vi "Main.vi"() -> ()   [LabVIEW 2013]
uses:
  <vilib>/myRIO/Instrument Drivers/Onboard IO/I2C/vis/Smart Open.vi
  <vilib>/myRIO/Instrument Drivers/Onboard IO/I2C/vis/Configure.vi
  <vilib>/myRIO/Instrument Drivers/Onboard IO/I2C/vis/Write Read.vi
  <vilib>/myRIO/Instrument Drivers/Onboard IO/I2C/vis/Write.vi
  <vilib>/myRIO/Instrument Drivers/Onboard IO/DIO/vis/Smart Open.vi
  <vilib>/myRIO/Instrument Drivers/Onboard IO/DIO/vis/Read.vi
  <vilib>/myRIO/Instrument Drivers/Onboard IO/I2C/vis/Read.vi
  <vilib>/myRIO/Common/Instrument Driver Framework/myRIO v1.0/UART/vis/myRIO v1.0 Close UART.vi
  <vilib>/myRIO/Instrument Drivers/Onboard IO/I2C/vis/Open.vi
  <vilib>/myRIO/Instrument Drivers/Onboard IO/DIO/vis/Open.vi
  <vilib>/myRIO/Common/Instrument Driver Framework/myRIO v1.0/I2C/vis/myRIO v1.1 Open I2C.vi
  <vilib>/myRIO/Common/Instrument Driver Framework/myRIO v1.0/DIO/vis/myRIO v1.1 Open DIO.vi
  <vilib>/myRIO/Common/Instrument Driver Framework/Utilities/vis/Validate Channels.vi
  <vilib>/myRIO/Common/Instrument Driver Framework/myRIO v1.0/I2C/vis/myRIO v1.0 Reserve I2C.vi
  <vilib>/myRIO/Common/Instrument Driver Framework/myRIO v1.0/DIO/vis/myRIO v1.0 Reserve DIO.vi
  <vilib>/myRIO/Common/Instrument Driver Framework/myRIO v1.0/I2C/vis/myRIO v1.0 Build MUX Configuration I2C.vi
  <vilib>/myRIO/Common/Instrument Driver Framework/myRIO v1.0/Resource Manager/vis/myRIO v1.0 Reserve Channel List.vi
  <vilib>/myRIO/Common/Instrument Driver Framework/myRIO v1.0/DIO/vis/myRIO v1.0 Build MUX Configuration DIO.vi
  <vilib>/myRIO/Common/Instrument Driver Framework/myRIO v1.0/Resource Manager/vis/myRIO v1.0 Create Configuration List.vi
  <vilib>/myRIO/Common/Instrument Driver Framework/myRIO v1.0/Resource Manager/vis/myRIO v1.0 Reserve Channel.vi
  <vilib>/myRIO/Common/Instrument Driver Framework/myRIO v1.0/Resource Manager/vis/myRIO v1.0 Unreserve Channel.vi
  <vilib>/myRIO/Common/Instrument Driver Framework/myRIO v1.0/Resource Manager/vis/myRIO v1.0 Build Mutex Name.vi
  <vilib>/myRIO/Common/Instrument Driver Framework/myRIO v1.0/myRIO v1.1 Open.vi
  <vilib>/Utility/VariantDataType/GetNumericInfo.vi
  <vilib>/Utility/error.llb/Error Cluster From Error Code.vi
  <vilib>/myRIO/Common/Instrument Driver Framework/Utilities/vis/IO Manager.vi
  <vilib>/myRIO/Common/Instrument Driver Framework/Utilities/vis/Configuration Manager.vi
  <vilib>/myRIO/Common/Instrument Driver Framework/myRIO v1.0/Resource Manager/vis/myRIO v1.0 Configure IO.vi
  <vilib>/myRIO/Common/Instrument Driver Framework/myRIO v1.0/myRIO v1.0 Close.vi
  <vilib>/myRIO/Common/Instrument Driver Framework/myRIO v1.0/I2C/vis/myRIO v1.0 Configure I2C.vi
  <vilib>/myRIO/Common/Instrument Driver Framework/myRIO v1.0/I2C/vis/myRIO v1.0 Write I2C.vi
  <vilib>/myRIO/Common/Instrument Driver Framework/myRIO v1.0/I2C/vis/myRIO v1.0 Read I2C.vi
  <vilib>/myRIO/Common/Instrument Driver Framework/myRIO v1.0/DIO/vis/myRIO v1.0 Read DIO.vi
  <vilib>/myRIO/Common/Instrument Driver Framework/Utilities/vis/FPGA Ref Manager.vi
  <vilib>/myRIO/Common/Instrument Driver Framework/myRIO v1.0/myRIO v1.0 Reset FPGA.vi
  <vilib>/myRIO/Instrument Drivers/Utilities/Utilities.lvlib
panel:
  out "Thyst (hysteresis)":u8[](array[numeric]) format="%02x"
  out "Tset (limit set)":u8[](array[numeric]) format="%02x"
  out "Config":u8[](array[numeric]) format="%08b"
  out "alert":bool
  out "temperature [ºC]":dbl(slide) scale=20.0..30.0
  out "Ta (ambient temp)":u8[](array[numeric]) format="%02x"
  in  "[ESC]":bool
  # "Temperature Sensor demo"
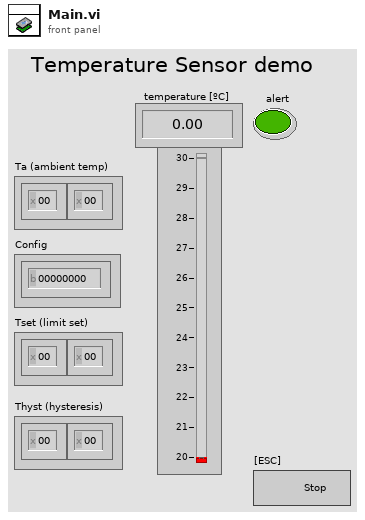
[diagram p1: front panel]
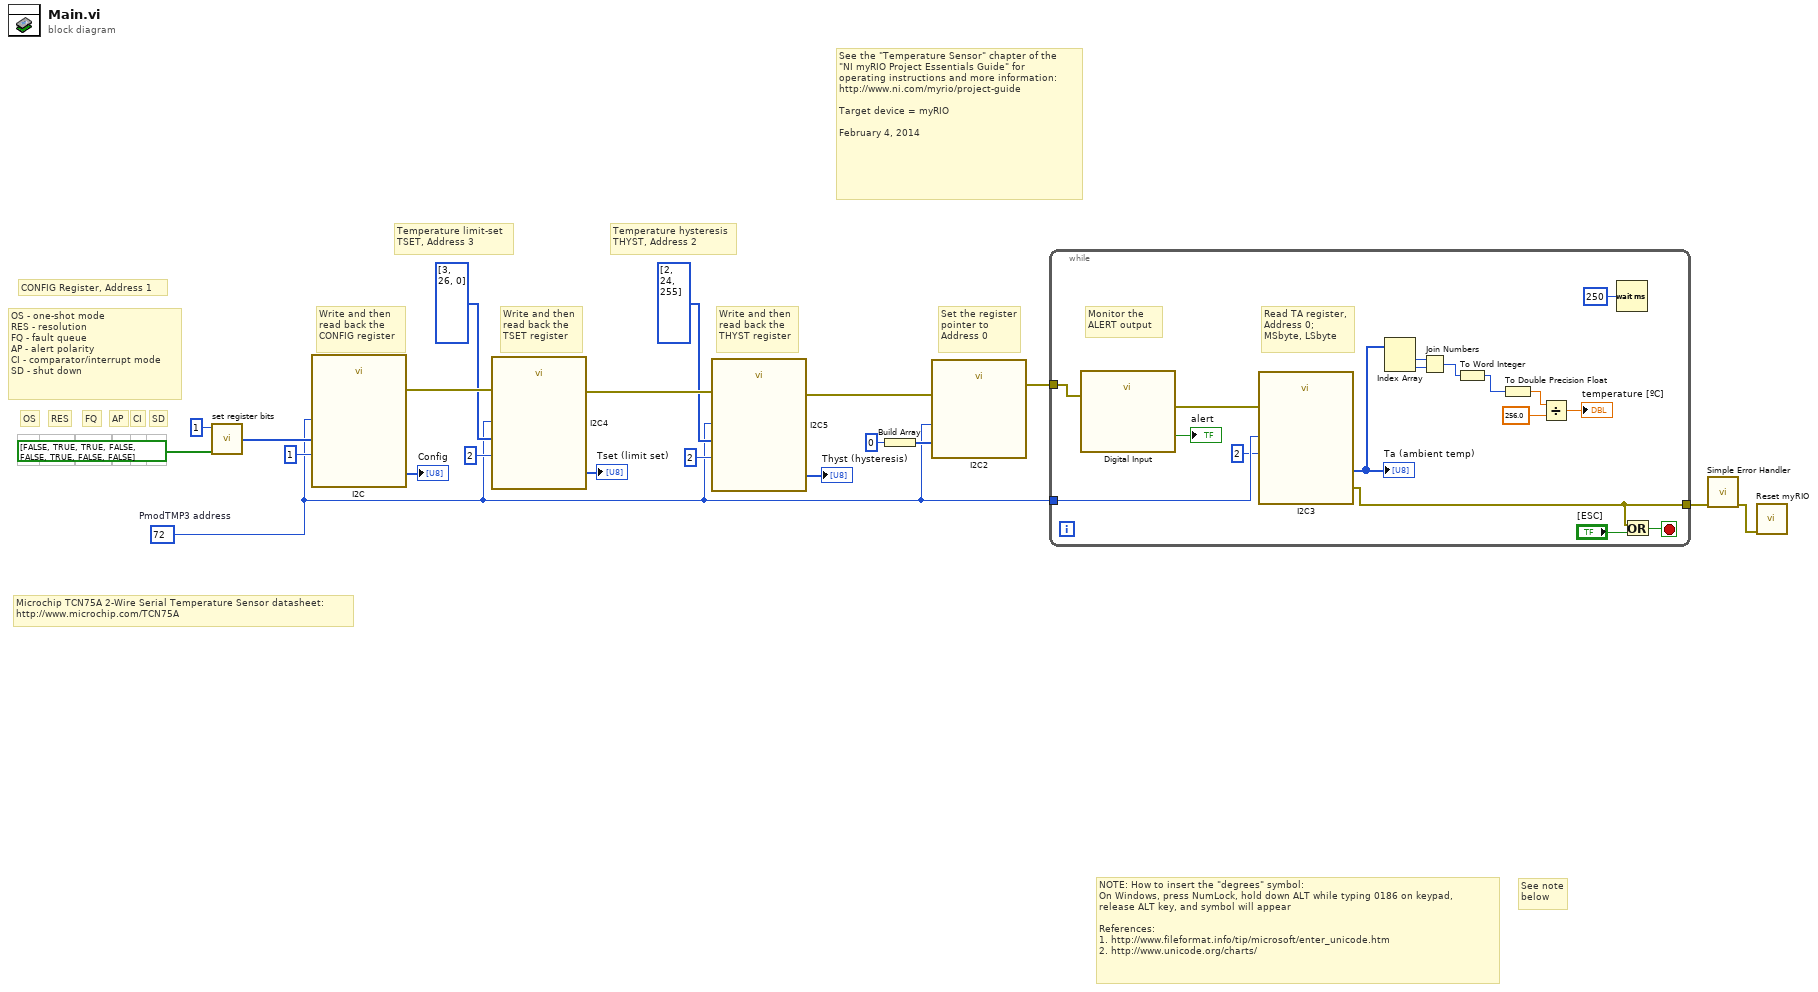
[diagram p0: block diagram]
diagram:
  w1 = u8 72  # PmodTMP3 address
  # "See the \"Temperature Sensor\" chapter of the\n\"NI myRIO Project Essentials Guide\" for\noperating instructions and more information: \nhttp://www.ni.com/myrio/project-guide\n\nTarget device = myRIO\n\nFebruary 4, 2014"
  # "Microchip TCN75A 2-Wire Serial Temperature Sensor datasheet:\nhttp://www.microchip.com/TCN75A"
  # "See note\nbelow"
  # "Write and then\nread back the\nCONFIG register"
  # "Write and then\nread back the\nTHYST register"
  # "Write and then\nread back the\nTSET register"
  # "Set the register\npointer to\nAddress 0"
  # "Temperature hysteresis\nTHYST, Address 2"
  # "Temperature limit-set\nTSET, Address 3"
  # "OS - one-shot mode\nRES - resolution\nFQ - fault queue\nAP - alert polarity\nCI - comparator/interrupt mode\nSD - shut down"
  # "SD"
  # "CI"
  # "AP"
  # "FQ"
  # "RES"
  # "OS"
  # "CONFIG Register, Address 1"
  # "NOTE: How to insert the \"degrees\" symbol:\nOn Windows, press NumLock, hold down ALT while typing 0186 on keypad,\nrelease ALT key, and symbol will appear\n\nReferences:\n1. http://www.fileformat.info/tip/microsoft/enter_unicode.htm\n2. http://www.unicode.org/charts/"
  n1 = call "set register bits.vi"("address"=u8 1, "register bits"=bool[] [FALSE, TRUE, TRUE, FALSE, FALSE, TRUE, FALSE, FALSE]) -> ("address / value"=w11:u8[])  [unwired: 5 in]
  n2 = call "I2C"("Slave Address (7-bit)"=w1, "Bytes to Write"=w11, "Byte Count"=u32 1) -> ("Bytes Read"=→"Config":u8[], "error out"=w15:errorcluster)  [unwired: 23 in]
  n3 = call "I2C4"("Slave Address (7-bit)"=w1, "Bytes to Write"=u8[] [3, 26, 0], "Byte Count"=u32 2, "error in (no error)"=w15) -> ("Bytes Read"=→"Tset (limit set)":u8[], "error out"=w14:errorcluster)  [unwired: 22 in]
  n4 = call "I2C5"("Slave Address (7-bit)"=w1, "Bytes to Write"=u8[] [2, 24, 255], "Byte Count"=u32 2, "error in (no error)"=w14) -> ("Bytes Read"=→"Thyst (hysteresis)":u8[], "error out"=w2:errorcluster)  [unwired: 22 in]
  n5 = Build Array(u8 0 ("address")) -> (w3:u8[])
  n6 = call "I2C2"("Slave Address (7-bit)"=w1, "Bytes to Write"=w3, "error in (no error)"=w2) -> ("error out"=w18:errorcluster)  [unwired: 24 in]
  n7 = while {
    tunnel: [w21] -> w19
    tunnel: w1 -> [w24]
    tunnel: w18 -> [w23]
    stop <- w36 stop-if-true
    # "Monitor the\nALERT output"
    # "Read TA register,\nAddress 0;\nMSbyte, LSbyte"
    n8 = call "Digital Input"("error in (no error)"=w23) -> ("B/DIO0 (Pin 11)"=→"alert":bool, "error out"=w28:errorcluster)  [unwired: 25 in]
    n9 = call "I2C3"("Slave Address (7-bit)"=w24, "Byte Count"=u32 2, "error in (no error)"=w28) -> ("Bytes Read"=w25:u8[], "error out"=w21:errorcluster)  [unwired: 23 in]
    "Ta (ambient temp)" <- w25
    n10 = Index Array "Index Array"(array=w25) -> (element #1=w32:u8, element #2=w31:u8)  [unwired: 2 in]
    n11 = Join Numbers(hi=w32, lo=w31) -> ((hi.lo)=w27:u16)
    n12 = To Word Integer(number=w27) -> (16bit integer=w26:i16)
    n13 = To Double Precision Float(number=w26) -> (double precision float=w34:dbl)
    n14 = Divide(x=w34, y=256.0) -> (x/y=→"temperature [ºC]":dbl)
    n15 = Wait (ms)(milliseconds to wait=u32 250) -> ()  [unwired: 1 out]
    n16 = Or(x=w21, y="[ESC]") -> (x .or. y?=w36:bool)
  }
  n17 = call <vilib>:"Simple Error Handler.vi"("error in (no error)"=w19) -> ("error out"=w20:errorcluster)  [unwired: 4 in, 4 out]
  n18 = call <vilib>:"Reset myRIO.vi"("error in (no error)"=w20) -> ()  [unwired: 10 in, 1 out]
